vi "Get Data Type of Python String Data.vi"(8 "error in (no error)":errorcluster, 10 "Python String":string) -> (0 "error out":errorcluster, 2 "data type":T1 format="%.0x")   [LabVIEW 2020, in "jki_python_data_tools.lvlib"]
uses:
  jki_python_data_tools.lvlib
  <userlib>/_OpenG.lib/lvdata/lvdata.llb/Type Descriptor Enumeration__ogtk.ctl
  <vilib>/regexp/Match Regular Expression.xnode
  <userlib>/_OpenG.lib/lvdata/lvdata.llb/openg_variant.lvlib
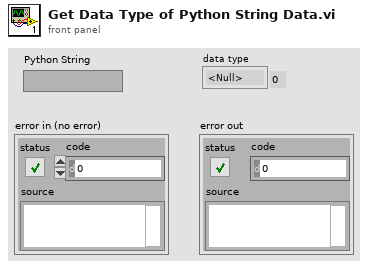
[diagram p1: front panel]
types:
  T1 = typedef "openg_variant.lvlib/Type Descriptor Enumeration__ogtk.ctl" = enum8{"<Null>", "I8", "I16", "I32", "I64", "U8", "U16", "U32", "U64", "SGL", "DBL", "EXT", "CSG", "CDB", "CXT", "0x0F", "0x10", "0x11", "0x12", "0x13", "0x14", "Enum U8", "Enum U16", "Enum U32", "Enum U64", "SGL PQ", "DBL PQ", "EXT PQ", "CSG PQ", "CDB PQ", "CXT PQ", "0x1F", "0x20", "Boolean", "0x22", "0x23", "0x24", "0x25", "0x26", "0x27", "0x28", "0x29", "0x2A", "0x2B", "0x2C", "0x2D", "0x2E", "0x2F", "String", "0x31", "Path", "Pict", "0x34", "0x35", "0x36", "DAQ", "0x38", "0x39", "0x3A", "0x3B", "0x3C", "0x3D", "0x3E", "0x3F", "Array", "0x41", "0x42", "0x43", "0x44", "0x45", "0x46", "0x47", "0x48", "0x49", "0x4A", "0x4B", "0x4C", "0x4D", "0x4E", "0x4F", "Cluster", "0x51", "0x52", "Variant", "Waveform", "0x55", "0x56", "0x57", "0x58", "0x59", "0x5A", "0x5B", "0x5C", "0x5D", "0x5E", "Fixed Point", "0x60", "0x61", "0x62", "0x63", "0x64", "0x65", "0x66", "0x67", "0x68", "0x69", "0x6A", "0x6B", "0x6C", "0x6D", "0x6E", "0x6F", "Refnum", "0x71", "0x72", "Set Collection", "Map Collection"}
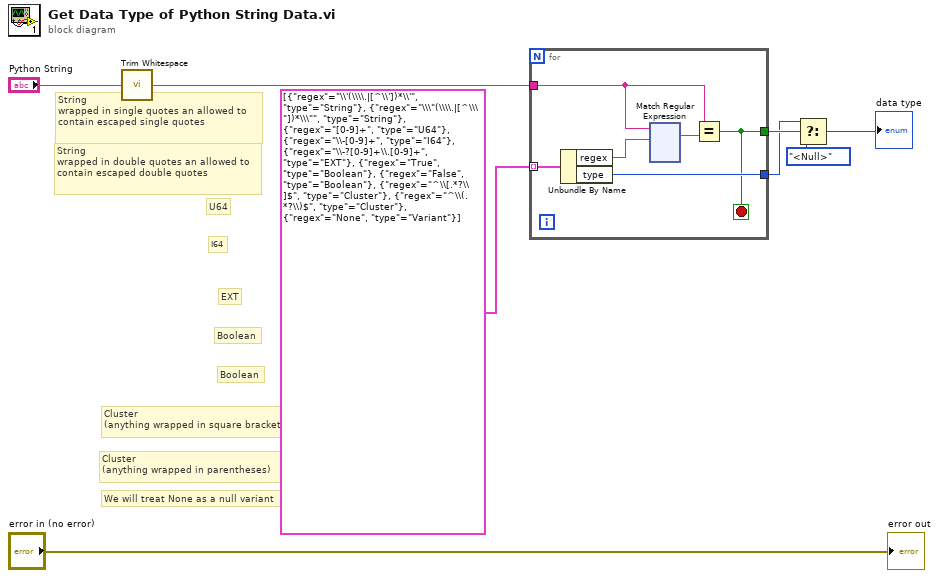
[diagram p0: block diagram]
diagram:
  # "We will treat None as a null variant"
  # "String\nwrapped in double quotes an allowed to contain escaped double quotes"
  # "Cluster\n(anything wrapped in parentheses)"
  # "Cluster\n(anything wrapped in square brackets)"
  # "Boolean"
  # "Boolean"
  # "EXT"
  # "I64"
  # "U64"
  # "String\nwrapped in single quotes an allowed to contain escaped single quotes"
  n1 = call <vilib>:"Trim Whitespace.vi"("string"="Python String") -> ("trimmed string"=w1:string)  [unwired: 1 in]
  n2 = for {
    tunnel: w1 -> [w11]
    tunnel: cluster{"regex":string, "type":T1}[] [{"regex"="\\'(\\\\.|[^\\'])*\\'", "type"=enum."String"}, {"regex"="\\\"(\\\\.|[^\\\"])*\\\"", "type"=enum."String"}, {"regex"="[0-9]+", "type"=enum."U64"}, {"regex"="\\-[0-9]+", "type"=enum."I64"}, {"regex"="\\-?[0-9]+\\.[0-9]+", "type"=enum."EXT"}, {"regex"="True", "type"=enum."Boolean"}, {"regex"="False", "type"=enum."Boolean"}, {"regex"="^\\[.*?\\]$", "type"=enum."Cluster"}, {"regex"="^\\(.*?\\)$", "type"=enum."Cluster"}, {"regex"="None", "type"=enum."Variant"}] -> [w14] mode=indexing
    tunnel: [w10] -> w5
    tunnel: [w9] -> w6
    stop <- w9 stop-if-true
    n3 = Unbundle By Name(w14) -> ("regex"=w13:string, "type"=w10:T1)
    n4 = xnode "Match Regular Expression"("input string"=w11, "regular expression"=w13) -> ("whole match"=w12:string)  [unwired: 4 in, 4 out]
    n5 = Equal?(x=w11, y=w12) -> (x = y?=w9:bool)
  }
  n6 = Select(t=w5, s=w6, f=Type_Descriptor_Enumeration__ogtk."<Null>") -> (s? t:f=→"data type":T1)
  "error out" <- "error in (no error)"
